vi "Construct.vi"(8 "port":i32, 9 "ReceiveTimeOut":i32, 10 "ConnectTimeOut":i32, 11 "ipAddress":string) -> (3 "MelsecMcNet out":refnum<class "MelsecMcNet.lvclass">)   [LabVIEW 2020, in "MelsecMcNet.lvclass"]
uses:
  MelsecMcNet.lvclass
  MelsecMcNet.lvclass/MelsecMcNet.ctl
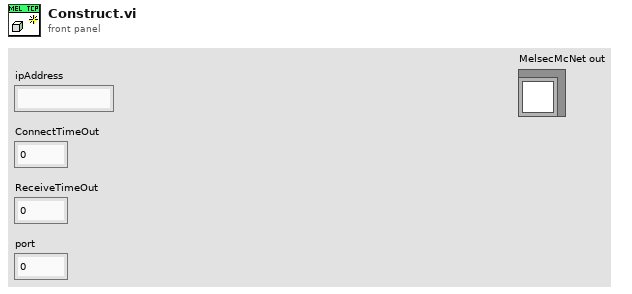
[diagram p1: front panel]
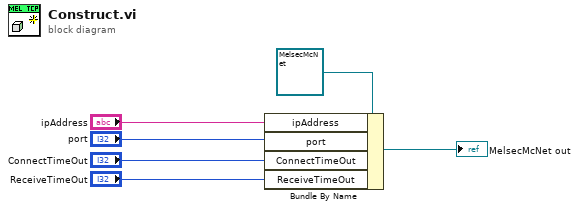
[diagram p0: block diagram]
diagram:
  n1 = Bundle By Name(cluster=refnum<class "MelsecMcNet.lvclass"> refnum ("MelsecMcNet in"), "ipAddress"="ipAddress", "port"="port", "ConnectTimeOut"="ConnectTimeOut", "ReceiveTimeOut"="ReceiveTimeOut") -> (→"MelsecMcNet out":refnum<class "MelsecMcNet.lvclass">)
